vi "Flat_seq.vi"() -> ()   [LabVIEW 2019]
panel:
  in  "Czas odniesienia":bool
  out "?":bool
  out "?":bool
  out "?":bool
  out "?":bool
  out "?":bool
  out "?":bool
  in  "?":bool
  out "Start 3. ramki [s]":dbl format="%.3f"
  out "Start 2. ramki [s]":dbl format="%.3f"
  out "Start 1. ramki [s]":dbl format="%.3f"
  in  "Trwanie 3. ramki [s]":dbl=1.0 caption="Delay Time (s)" min=0.0 step=0.2
  in  "Trwanie 2. ramki [s]":dbl=1.0 caption="Delay Time (s)" min=0.0 step=0.2
  in  "Trwanie 1. ramki [s]":dbl=1.0 caption="Delay Time (s)" min=0.0 step=0.2
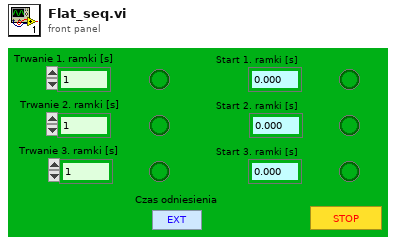
[diagram p1: front panel]
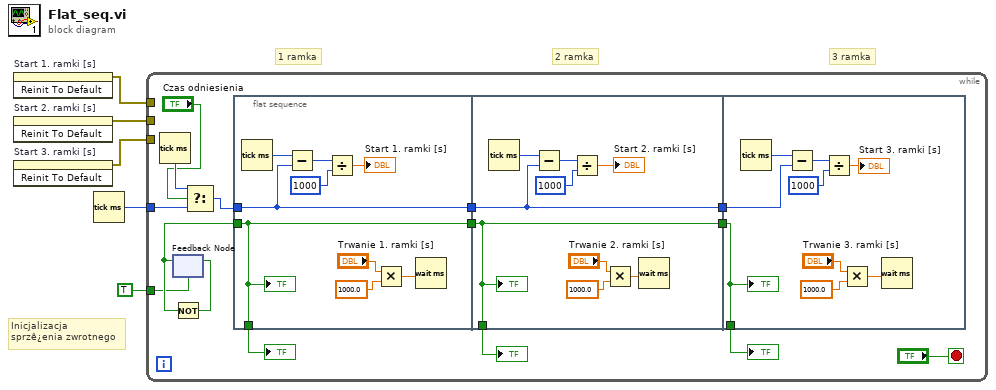
[diagram p0: block diagram]
diagram:
  # "Inicjalizacja\nsprzê¿enia zwrotnego"
  # "3 ramka"
  # "2 ramka"
  # "1 ramka"
  n1 = invoke on="Start 1. ramki [s]" class="DigNum (strict)" method="Reinit To Default"() -> (error out=w4:errorcluster)  [unwired: 3 in, 2 out]
  n2 = invoke on="Start 2. ramki [s]" class="DigNum (strict)" method="Reinit To Default"() -> (error out=w3:errorcluster)  [unwired: 3 in, 2 out]
  n3 = invoke on="Start 3. ramki [s]" class="DigNum (strict)" method="Reinit To Default"() -> (error out=w2:errorcluster)  [unwired: 3 in, 2 out]
  n4 = Tick Count (ms)() -> (millisecond timer value=w1:u32)
  n5 = while {
    tunnel: w1 -> [w8]
    tunnel: TRUE -> [w10]
    tunnel: w4 -> [_]
    tunnel: w3 -> [_]
    tunnel: w2 -> [_]
    stop <- "?" stop-if-true
    n6 = Tick Count (ms)() -> (millisecond timer value=w9:u32)
    n7 = feedback #1(w10) -> (w18:bool)
    n8 = Not(x=w18) -> (.not. x?=w19:bool)
    n9 = feedback-in #1(w19) -> ()
    n10 = Select(t=w9, s="Czas odniesienia", f=w8) -> (s? t:f=w7:u32)
    n11 = flat-sequence {
      tunnel: w18 -> [w29]
      tunnel: [w29] -> w14
      tunnel: [w29] -> w17
      tunnel: w7 -> [w27]
      tunnel: [w27] -> w12
      tunnel: w14 -> [w38]
      tunnel: [w38] -> w13
      tunnel: [w38] -> w16
      tunnel: w12 -> [w36]
      tunnel: [w36] -> w11
      tunnel: w13 -> [w47]
      tunnel: [w47] -> w15
      tunnel: w11 -> [w45]
      frame #0 {
        n12 = Tick Count (ms)() -> (millisecond timer value=w28:u32)
        n13 = Subtract(x=w28, y=w27) -> (x-y=w25:u32)
        n14 = Divide(x=w25, y=u32 1000) -> (x/y=→"Start 1. ramki [s]":dbl)
        n15 = Multiply(x="Trwanie 1. ramki [s]", y=1000.0) -> (x*y=w23:dbl)
        n16 = Wait (ms)(milliseconds to wait=w23) -> ()  [unwired: 1 out]
        "?" <- w29
      }
      frame #1 {
        n17 = Tick Count (ms)() -> (millisecond timer value=w37:u32)
        n18 = Subtract(x=w37, y=w36) -> (x-y=w34:u32)
        n19 = Divide(x=w34, y=u32 1000) -> (x/y=→"Start 2. ramki [s]":dbl)
        n20 = Multiply(x="Trwanie 2. ramki [s]", y=1000.0) -> (x*y=w32:dbl)
        n21 = Wait (ms)(milliseconds to wait=w32) -> ()  [unwired: 1 out]
        "?" <- w38
      }
      frame #2 {
        n22 = Tick Count (ms)() -> (millisecond timer value=w46:u32)
        n23 = Subtract(x=w46, y=w45) -> (x-y=w42:u32)
        n24 = Divide(x=w42, y=u32 1000) -> (x/y=→"Start 3. ramki [s]":dbl)
        n25 = Multiply(x="Trwanie 3. ramki [s]", y=1000.0) -> (x*y=w41:dbl)
        n26 = Wait (ms)(milliseconds to wait=w41) -> ()  [unwired: 1 out]
        "?" <- w47
      }
    }
    "?" <- w17
    "?" <- w16
    "?" <- w15
  }
